vi "Initialise.vi"(8 "error in (no error)":errorcluster, 10 "System In":refnum<class "abs_System.lvclass">, 11 "Node in":refnum<class "abs_Node.lvclass">) -> (0 "error out":errorcluster, 2 "System Out":refnum<class "abs_System.lvclass">, 3 "Node out":refnum<class "abs_Node.lvclass">)   [LabVIEW 2021, in "BT.lvlib" / "abs_Node.lvclass"]
uses:
  abs_Node.lvclass
  abs_System/abs_System.lvclass
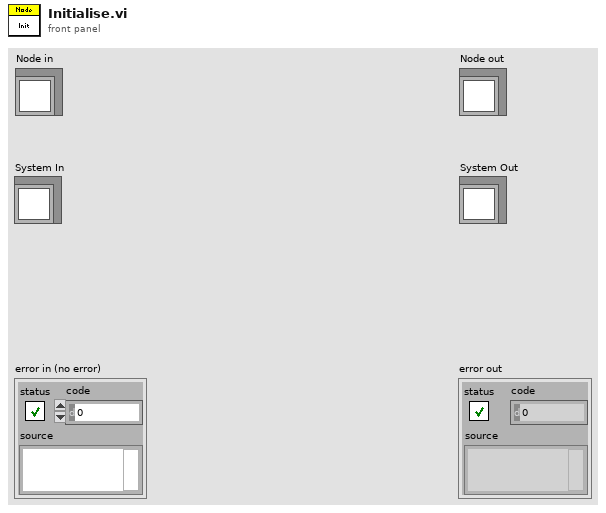
[diagram p1: front panel]
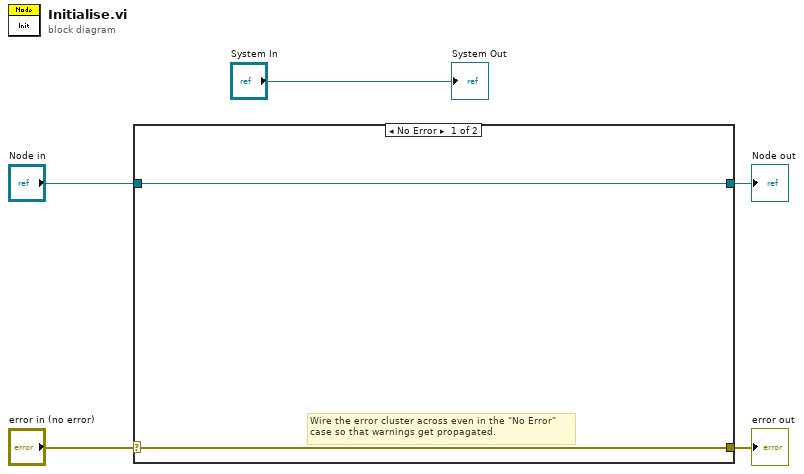
[diagram p0: block diagram]
diagram:
  n1 = case shown="No Error" "error in (no error)" {
    selector: "error in (no error)" -> [w6 w9]
    tunnel: [w6 w9] -> w4
    tunnel: [w7 w8] -> w2
    tunnel: "Node in" -> [w7 w8]
    frame No Error {
      # "Wire the error cluster across even in the \"No Error\"\ncase so that warnings get propagated."
    }
    frame Error {
    }
  }
  "error out" <- w4
  "Node out" <- w2
  "System Out" <- "System In"
